vi "Get UIPs.vi"(8 "Error In":errorcluster, 11 "UIM In":refnum<data-value>) -> (0 "Error Out":errorcluster, 1 "Enabled":bool[](array[boolean]), 2 "UIPs":refnum<class "UIP.lvclass">[](array[class]), 3 "UIM Out":refnum<data-value>)   [LabVIEW 2015, in "UIM.lvclass"]
doc: "List all UIPs currently loaded and used by the UIM. The flag output provides information if th UIP is enabled."
uses:
  UIM.lvclass
  UIP/UIP.lvclass
  UIM.lvclass/UIM.ctl
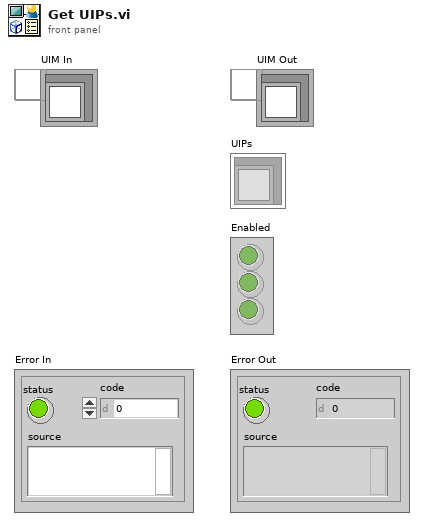
[diagram p1: front panel]
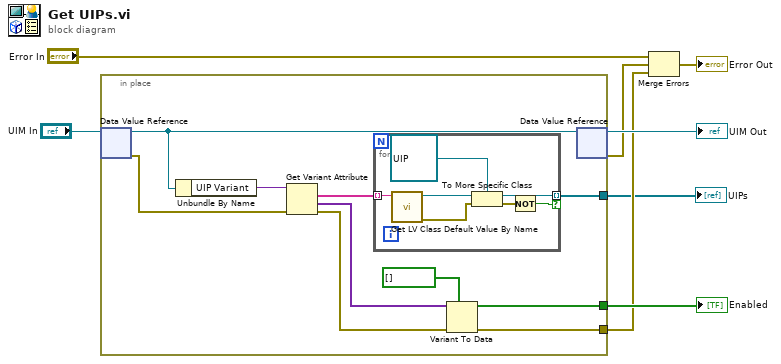
[diagram p0: block diagram]
diagram:
  n1 = in-place {
    in-place-border: [w16] -> w3
    in-place-border: [w15] -> w6
    in-place-border: [w9] -> w1
    n2 = in-place-dvr #1("UIM In") -> (w18:refnum<class "UIM.lvclass">, w10:errorcluster)
    n3 = Unbundle By Name(w18) -> ("UIP Variant"=w14:variant)
    n4 = Get Variant Attribute(Variant=w14, error in=w10) -> (names=w13:string[], values=w12:variant[], error out=w11:errorcluster)  [unwired: 2 in, 1 out]
    n5 = for {
      tunnel: w13 -> [w25] mode=indexing
      tunnel: [w21] -> w9 mode=indexing if=w19
      n6 = call <vilib>:"Get LV Class Default Value By Name.vi"("class name"=w25) -> ("error out"=w22:errorcluster, "object"=w24:refnum<class>)  [unwired: 9 in]
      n7 = To More Specific Class(target class=refnum<class "UIP.lvclass"> refnum ("UIP"), reference=w24, error in=w22) -> (specific class reference=w21:refnum<class "UIP.lvclass">, error out=w20:errorcluster)
      n8 = Not(x=w20) -> (.not. x?=w19:bool)
    }
    n9 = Variant To Data(error in=w11, type=bool[] [], Variant=w12) -> (data=w15:bool[], error out=w16:errorcluster)
    n10 = in-place-dvr #1(w18) -> (→"UIM Out":refnum<data-value>, w2:errorcluster)
  }
  "Enabled" <- w6
  "UIPs" <- w1
  n11 = Merge Errors("Error In", w2, w3) -> (→"Error Out":errorcluster)
